vi "Panic.vi"(11 "message (\"\")":string) -> ()   [LabVIEW 2024, in "Utilities.lvlib"]
uses:
  Utilities.lvlib
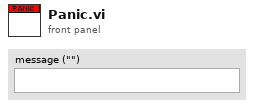
[diagram p1: front panel]
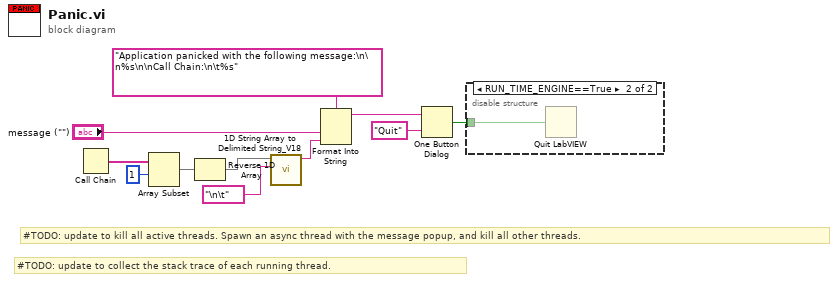
[diagram p0: block diagram]
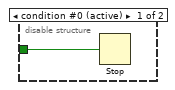
[diagram p2: hidden frame]
diagram:
  # "#TODO: update to collect the stack trace of each running thread."
  # "#TODO: update to kill all active threads. Spawn an async thread with the message popup, and kill all other threads."
  n1 = Call Chain() -> (call chain=w5:string[])
  n2 = Array Subset(array=w5, index=1) -> (w4:string[])  [unwired: 1 in]
  n3 = Reverse 1D Array(array=w4) -> (reversed array=w3:string[])
  n4 = call "1D String Array to Delimited String_V18.vi"("delimiter"="\n\t", "string array"=w3) -> ("delimited string"=w1:string)  [unwired: 9 in]
  n5 = Format Into String(format string="Application panicked with the following message:\n\n%s\n\nCall Chain:\n\t%s", "message (\"\")", w1) -> (resulting string=w7:string)  [unwired: 2 in, 1 out]
  n6 = One Button Dialog(message=w7, button name ("OK")="Quit") -> (true=w11:bool)
  n7 = disable-structure shown="RUN_TIME_ENGINE==True" {
    disable-tunnel: w11 -> [w12 w13]
    frame condition #0 (active) {
      n8 = Stop(stop? (T)=w12) -> ()
    }
    frame condition #1 {
      n9 = Quit LabVIEW(quit? (T)=w13) -> ()
    }
  }
